vi "Exercise1.17-Tick Count (ms).vi"() -> ()   [LabVIEW 2013]
uses:
  <vilib>/measure/NI_MABase.lvlib
panel:
  out "Waveform Graph":dbl[](graph)
  out "Count":i32
  out "Time elapsed":u32
  in  "stop":bool
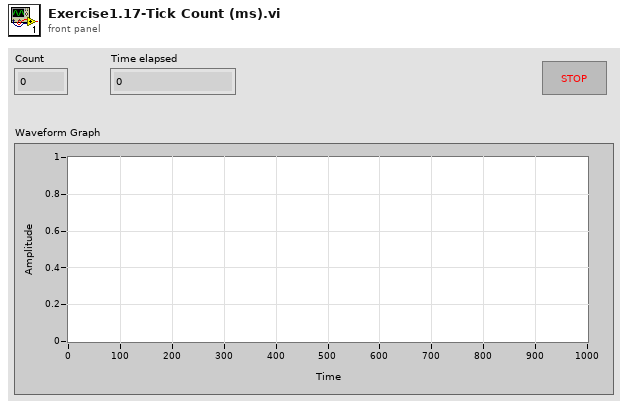
[diagram p1: front panel]
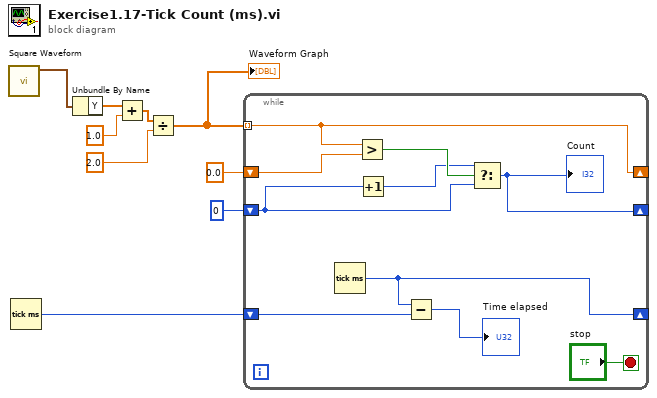
[diagram p0: block diagram]
diagram:
  n1 = call <vilib>:"Square Waveform.vi"() -> ("signal out"=w6:waveform(dbl))  [unwired: 10 in, 1 out]
  n2 = Tick Count (ms)() -> (millisecond timer value=w9:u32)
  n3 = Unbundle By Name(w6) -> ("Y"=w5:dbl[])
  n4 = Add(x=w5, y=1.0) -> (x+y=w3:dbl[])
  n5 = Divide(x=w3, y=2.0) -> (x/y=w1:dbl[])
  "Waveform Graph" <- w1
  n6 = while {
    shift-right: [w16] -> _
    shift-left: w9 -> [w19]
    shift-right: [w13] -> _
    shift-left: 0.0 -> [w15]
    tunnel: w1 -> [w13] mode=indexing
    shift-right: [w12] -> _
    shift-left: 0 -> [w10]
    stop <- "stop" stop-if-true
    n7 = Tick Count (ms)() -> (millisecond timer value=w16:u32)
    n8 = Greater?(x=w13, y=w15) -> (0:w14:bool)
    n9 = Increment(x=w10) -> (x+1=w11:i32)
    n10 = Subtract(x=w16, y=w19) -> (x-y=→"Time elapsed":u32)
    n11 = Select(t=w11, s=w14, f=w10) -> (s? t:f=w12:i32)
    "Count" <- w12
  }
